vi "read_conf.vi"() -> (1 "Seuil":dbl, 2 "TCPU":dbl)   [LabVIEW 2019]
uses:
  <vilib>/Utility/config.llb/Read Key (Double).vi
  <vilib>/Utility/config.llb/Read Key (U32).vi
  <vilib>/Utility/config.llb/NI_LVConfig.lvlib
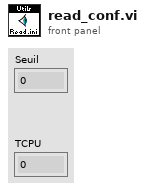
[diagram p1: front panel]
types:
  T1 = typedef "NI_LVConfig.lvlib/Config Data RefNum.ctl" = refnum<k1>
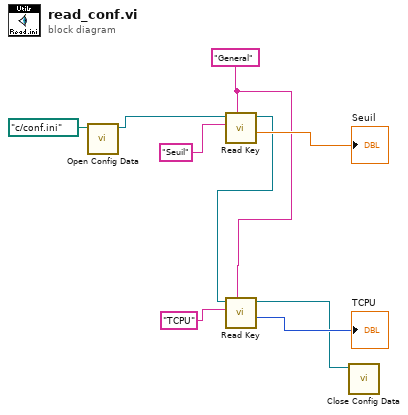
[diagram p0: block diagram]
diagram:
  w2 = "General" ("section")
  n1 = call <vilib>:"Open Config Data.vi"("configuration file path"=path "c:/conf.ini") -> ("refnum"=w4:T1)  [unwired: 8 in, 2 out]
  n2 = call-poly <vilib>:"Read Key.vi"("section"=w2, "key"="Seuil", "refnum"=w4) -> ("value"=→"Seuil":dbl, "refnum out"=w3:T1)  [unwired: 5 in, 2 out]
  n3 = call-poly <vilib>:"Read Key.vi"("section"=w2, "key"="TCPU", "refnum"=w3) -> ("value"=→"TCPU":u32, "refnum out"=w1:T1)  [unwired: 5 in, 2 out]
  n4 = call <vilib>:"Close Config Data.vi"("refnum"=w1) -> ()  [unwired: 9 in, 2 out]
